vi "Ft_To_Inches.vi"(10 "Ft":dbl) -> (2 "In":dbl)   [LabVIEW 2012]
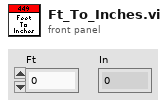
[diagram p1: front panel]
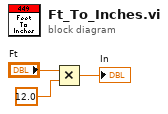
[diagram p0: block diagram]
diagram:
  n1 = Multiply(x="Ft", y=12.0) -> (x*y=→"In":dbl)
